vi "Vbias Word To dB.vi"(0 "Vbias Word":u8 format="%08b") -> (4 "dB":dbl)   [LabVIEW 2020]
uses:
  <vilib>/gmath/NI_Gmath.lvlib
  7a608241-77eb-4d9e-a402-85fb6f76b42e.vi
panel:
  in  "Vbias Word 2":u8=7 format="%08b"
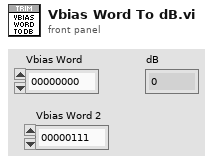
[diagram p1: front panel]
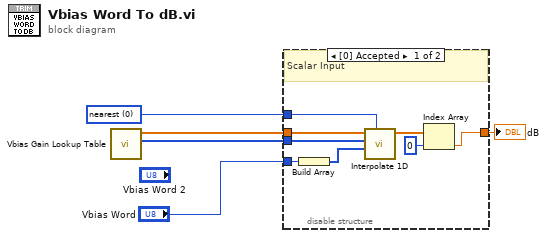
[diagram p0: block diagram]
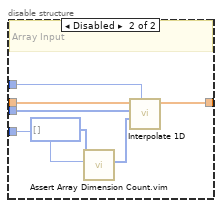
[diagram p2: hidden frame]
diagram:
  w5 = 0 items=["nearest", "linear", "spline", "cubic Hermite", "Lagrange"] ("method")
  n1 = call "Vbias Gain Lookup Table.vi"() -> ("ROUT<7:5>"=w4:u8[], "VB Gain(dB)"=w3:dbl[])  [unwired: 10 in]
  n2 = disable-structure shown="[0] Accepted" {
    disable-tunnel: w5 -> [w13 w20]
    disable-tunnel: w4 -> [w12 w19]
    disable-tunnel: w3 -> [w11 w18]
    disable-tunnel: [w7 w17] -> w2
    disable-tunnel: "Vbias Word" -> [w10 w15]
    frame Enabled {
      # "Scalar Input"
      n3 = Build Array(w10) -> (w9:u8[])
      n4 = call <vilib>:"Interpolate 1D.vi"("method"=w13, "xi"=w9, "X"=w12, "Y"=w11) -> ("yi"=w8:dbl[])  [unwired: 5 in, 2 out]
      n5 = Index Array(array=w8, index=0) -> (element=w7:dbl)
    }
    frame Disabled {
      # "Array Input"
      n6 = call "Assert Array Dimension Count.vim"("array type"=u8[] [], "value in"=w15) -> ("value out"=w14:u8[])  [unwired: 7 in]
      n7 = call <vilib>:"Interpolate 1D.vi"("method"=w20, "xi"=w14, "X"=w19, "Y"=w18) -> ("yi"=w17:dbl[])  [unwired: 5 in, 2 out]
    }
  }
  "dB" <- w2
